vi "NullArray_I.vi"() -> (3 "Null Array":i32[](array[numeric]))   [LabVIEW 2013]
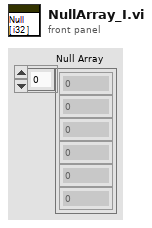
[diagram p1: front panel]
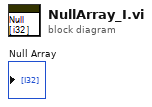
[diagram p0: block diagram]
diagram:
